vi "merge_One Shot Falling With Input.vi"   [LabVIEW 2020, in "NI_FunctionBlockMergeVIs.lvlib"]
doc: "Detects a falling edge, a transition from TRUE to FALSE, on the input signal. When a falling edge occurs, <B>output</B> is TRUE for one function block execution. The value of <B>output</B> remains FALSE until a new falling edge occurs."
uses:
  <vilib>/functionblocks/NI_FunctionBlockMergeVIs.lvlib
  <vilib>/functionblocks/FB Core/FB Core.xnode
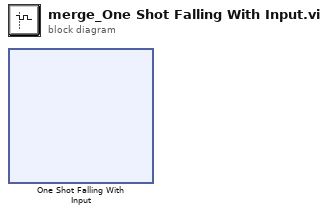
[diagram p0: block diagram]
diagram:
  n1 = xnode "One Shot Falling With Input"() -> ()  [unwired: 2 in, 2 out]
